vi "Pressure_Multiplexer_Server_Global.vi"() -> ()   [LabVIEW 2020]
uses:
  Controls/Setup.ctl
  Controls/Trigger_Mode.ctl
panel:
  in  "Acquisition Rendezvous Server":T1
  in  "Time per Block (s)":dbl=100.0 format="%_4f"
  in  "Trigger mode":T2
  in  "setup":T3=enum."Show Setup"
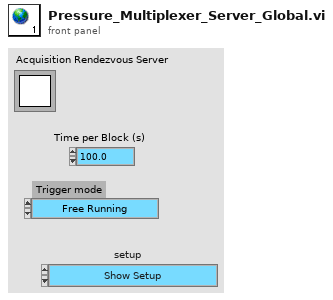
[diagram p1: front panel]
types:
  T1 = typedef "Rendezvous RefNum" = refnum<k1>
  T2 = typedef "Trigger_Mode.ctl" = enum16{"Free Running", "Start on Trigger", "Trigger Every Block", "Trigger Every Sample"}
  T3 = typedef "Setup.ctl" = enum16{"Run Program", "Show Setup", "Save Current Setup", "Setup Front Panel"}
diagram:
